vi "Edit.vi"(11 "TS.SequenceContext":refnum<k7>) -> (0 "error out":errorcluster)   [LabVIEW 2011]
panel:
  in  "Result":refnum<k7>(container)
  in  "Operator":enum16{"Add", "Divide", "Multiple", "Subtract"}(ring)
  in  "Number 2":refnum<k7>(container)
  in  "Number 1":refnum<k7>(container)
  out "Preview Result":dbl
  in  "OK":bool
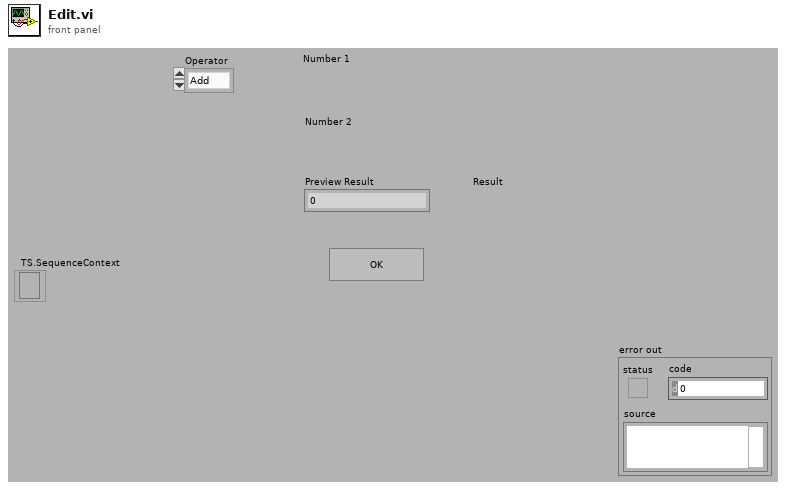
[diagram p1: front panel]
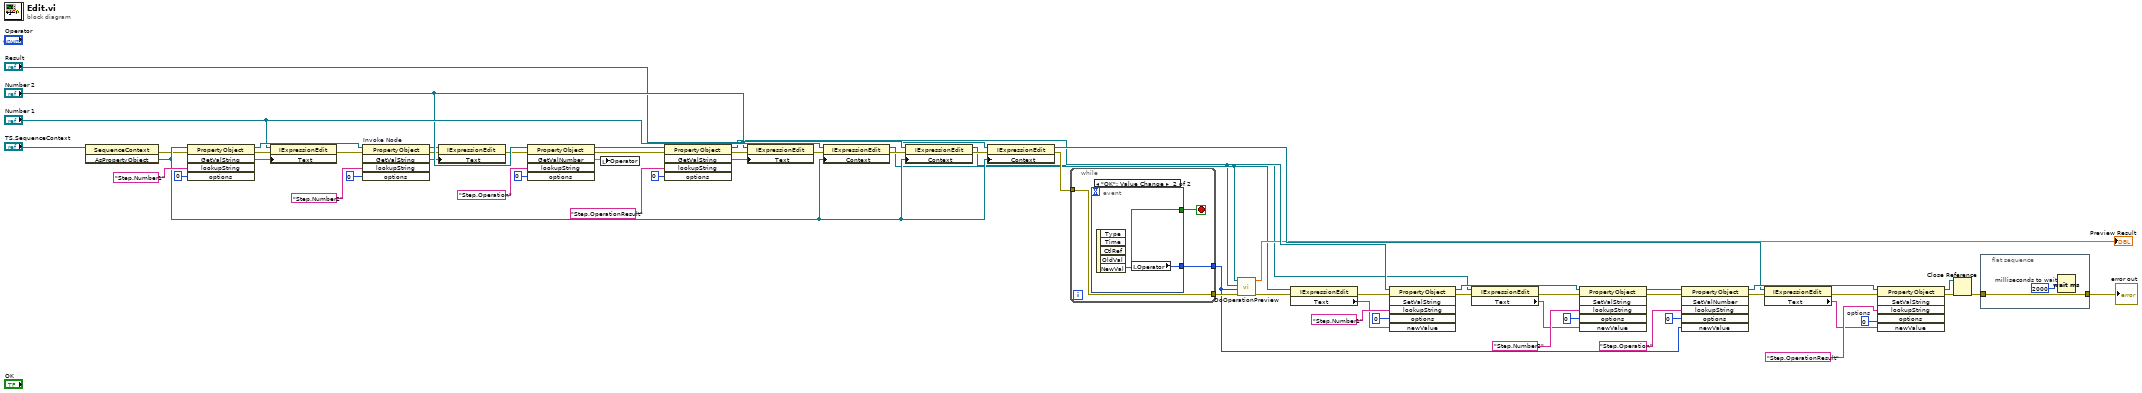
[diagram p0: block diagram]
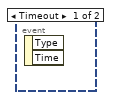
[diagram p2: hidden frame]
diagram:
  w50 = 0  # options
  n1 = invoke class="SequenceContext" method="AsPropertyObject"(reference="TS.SequenceContext") -> (error out=w20:errorcluster, "AsPropertyObject"=w33:refnum<k7>)  [unwired: 2 in, 1 out]
  n2 = invoke class="PropertyObject" method="GetValString"(reference=w33, error in=w20, "lookupString"="Step.Number1", "options"=0) -> (reference out=w36:refnum<k7>, error out=w19:errorcluster, "GetValString"=w18:string)  [unwired: 1 in, 2 out]
  n3 = property class="IExpressionEdit"(reference="Number 1", error in=w19, "Text"=w18) -> (error out=w15:errorcluster)  [unwired: 1 out]
  n4 = invoke on="Invoke Node" class="PropertyObject" method="GetValString"(reference=w36, error in=w15, "lookupString"="Step.Number2", "options"=0) -> (reference out=w35:refnum<k7>, error out=w16:errorcluster, "GetValString"=w17:string)  [unwired: 1 in, 2 out]
  n5 = property class="IExpressionEdit"(reference="Number 2", error in=w16, "Text"=w17) -> (error out=w14:errorcluster)  [unwired: 1 out]
  n6 = invoke class="PropertyObject" method="GetValNumber"(reference=w35, error in=w14, "lookupString"="Step.Operation", "options"=0) -> (reference out=w34:refnum<k7>, error out=w12:errorcluster, "GetValNumber"=w13:dbl)  [unwired: 1 in, 2 out]
  n7 = local write "Operator"(w13) -> ()
  n8 = invoke class="PropertyObject" method="GetValString"(reference=w34, error in=w12, "lookupString"="Step.OperationResult", "options"=0) -> (reference out=w26:refnum<k7>, error out=w11:errorcluster, "GetValString"=w10:string)  [unwired: 1 in, 2 out]
  n9 = property class="IExpressionEdit"(reference="Result", error in=w11, "Text"=w10) -> (error out=w9:errorcluster)  [unwired: 1 out]
  n10 = property class="IExpressionEdit"(reference="Number 1", error in=w9, "Context"=w33) -> (reference out=w5:refnum<k7>, error out=w62:errorcluster)
  n11 = property class="IExpressionEdit"(reference="Number 2", error in=w62, "Context"=w33) -> (reference out=w4:refnum<k7>, error out=w41:errorcluster)
  n12 = property class="IExpressionEdit"(reference="Result", error in=w41, "Context"=w33) -> (reference out=w40:refnum<k7>, error out=w25:errorcluster)
  n13 = while {
    tunnel: w25 -> [w65]
    tunnel: [w65] -> w8
    tunnel: [w64] -> w1
    stop <- w66 stop-if-true
    n14 = event shown="[1] \"OK\": Value Change" {
      selector: _ -> [_ _]
      dyn-events: _ -> [_ _]
      timeout: _ -> [_ _]
      tunnel: [_ w68] -> w66
      tunnel: [_ w67] -> w64
      event Timeout {
        n15 = event-data() -> ()  [unwired: 1 in, 2 out]
      }
      event "OK": Value Change {
        n16 = event-data() -> ("NewVal"=w68:bool)  [unwired: 1 in, 4 out]
        n17 = local read "Operator"() -> (w67:enum16{"Add", "Divide", "Multiple", "Subtract"})
      }
    }
  }
  n18 = call "DoOperationPreview.vi"("error in (no error)"=w8, "Operator"=w1, "TestStand UI ExpressionEdit Control 2"=w4, "TestStand UI ExpressionEdit Control"=w5) -> ("error out"=w7:errorcluster, "Result"=→"Preview Result":dbl)  [unwired: 6 in]
  n19 = property class="IExpressionEdit"(reference=w5, error in=w7) -> (error out=w46:errorcluster, "Text"=w48:string)  [unwired: 1 out]
  n20 = invoke class="PropertyObject" method="SetValString"(reference=w26, error in=w46, "lookupString"="Step.Number1", "options"=0, "newValue"=w48) -> (reference out=w60:refnum<k7>, error out=w45:errorcluster)  [unwired: 1 in, 4 out]
  n21 = property class="IExpressionEdit"(reference=w4, error in=w45) -> (error out=w44:errorcluster, "Text"=w47:string)  [unwired: 1 out]
  n22 = invoke class="PropertyObject" method="SetValString"(reference=w60, error in=w44, "lookupString"="Step.Number2", "options"=0, "newValue"=w47) -> (reference out=w58:refnum<k7>, error out=w57:errorcluster)  [unwired: 1 in, 4 out]
  n23 = invoke class="PropertyObject" method="SetValNumber"(reference=w58, error in=w57, "lookupString"="Step.Operation", "options"=0, "newValue"=w1) -> (reference out=w52:refnum<k7>, error out=w39:errorcluster)  [unwired: 1 in, 4 out]
  n24 = property class="IExpressionEdit"(reference=w40, error in=w39) -> (error out=w38:errorcluster, "Text"=w49:string)  [unwired: 1 out]
  n25 = invoke class="PropertyObject" method="SetValString"(reference=w52, error in=w38, "lookupString"="Step.OperationResult", "options"=w50, "newValue"=w49) -> (reference out=w42:refnum<k7>, error out=w43:errorcluster)  [unwired: 1 in, 4 out]
  n26 = Close Reference(reference=w42, error in (no error)=w43) -> (error out=w3:errorcluster)
  n27 = flat-sequence {
    tunnel: w3 -> [w70]
    tunnel: [w70] -> w2
    frame #0 {
      w69 = u32 2000  # milliseconds to wait
      n28 = Wait (ms)(milliseconds to wait=w69) -> ()  [unwired: 1 out]
    }
  }
  "error out" <- w2
